vi "QueryServer_Template.vi"() -> ()   [LabVIEW 2019]
panel:
  in  "stop":bool
  in  "Server Address":string
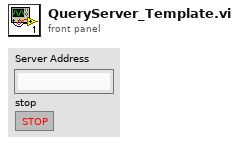
[diagram p1: front panel]
types:
  T1 = cluster{"event":refnum<user-event>, "event":refnum<user-event>, "event":refnum<user-event>}
  T2 = typedef "QueryServer_gRPCid.ctl" = cluster{"ID":u64}
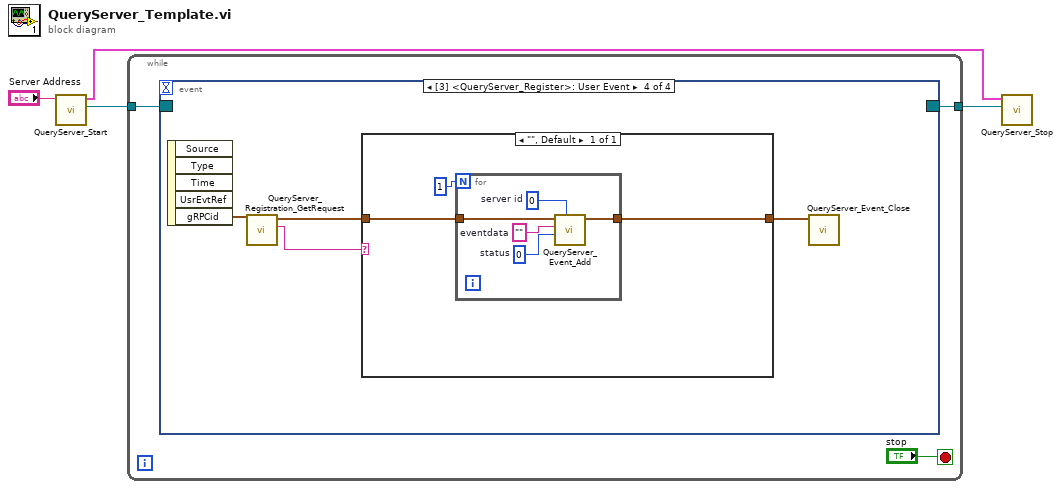
[diagram p0: block diagram]
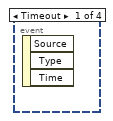
[diagram p2: hidden frame]
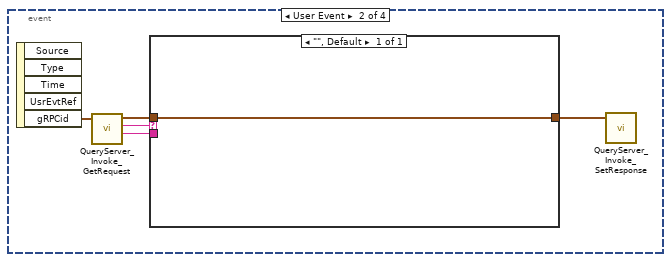
[diagram p3: hidden frame]
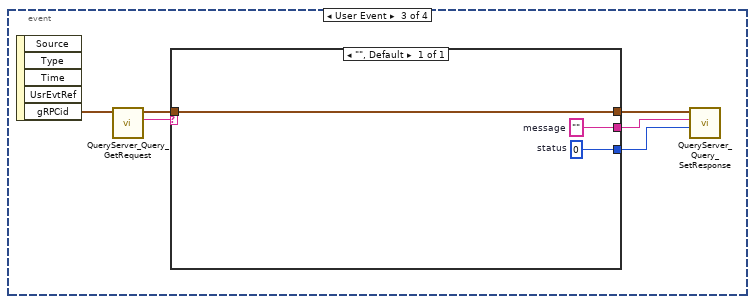
[diagram p4: hidden frame]
diagram:
  n1 = call "QueryServer_Start.vi"("Server Address"="Server Address") -> ("Event Registration Refnum"=w3:refnum<event-registration>, "Server Events"=w1:T1)  [unwired: 7 in, 1 out]
  n2 = while {
    tunnel: w3 -> [w6]
    tunnel: [w5] -> w2
    stop <- "stop" stop-if-true
    n3 = event shown="[3] <QueryServer_Register>: User Event" {
      selector: w6 -> [_ _ _ _]
      dyn-events: [_ _ _ _] -> w5
      timeout: _ -> [_ _ _ _]
      event Timeout {
        n4 = event-data() -> ()  [unwired: 1 in, 3 out]
      }
      event User Event {
        n5 = event-data() -> ("gRPCid"=w12:T2)  [unwired: 1 in, 4 out]
        n6 = call "QueryServer_Invoke_GetRequest.vi"("gRPCid"=w12) -> ("parameter"=w8:string, "command"=w11:string, "gRPCid out"=w10:T2)  [unwired: 5 in, 1 out]
        n7 = case shown="\"\", Default" w11 {
          tunnel: w10 -> [w13]
          tunnel: [w13] -> w9
          tunnel: w8 -> [_]
          frame "", Default {
          }
        }
        n8 = call "QueryServer_Invoke_SetResponse.vi"("gRPCid"=w9) -> ()  [unwired: 9 in, 1 out]
      }
      event User Event {
        n9 = event-data() -> ("gRPCid"=w19:T2)  [unwired: 1 in, 4 out]
        n10 = call "QueryServer_Query_GetRequest.vi"("gRPCid"=w19) -> ("gRPCid out"=w17:T2, "query"=w18:string)  [unwired: 7 in, 1 out]
        n11 = case shown="\"\", Default" w18 {
          tunnel: w17 -> [w22]
          tunnel: [w22] -> w16
          tunnel: [w21] -> w15
          tunnel: [w20] -> w14
          frame "", Default {
            w20 = 0  # status
            w21 = ""  # message
          }
        }
        n12 = call "QueryServer_Query_SetResponse.vi"("gRPCid"=w16, "message"=w15, "status"=w14) -> ()  [unwired: 7 in, 1 out]
      }
      event User Event {
        n13 = event-data() -> ("gRPCid"=w26:T2)  [unwired: 1 in, 4 out]
        n14 = call "QueryServer_Registration_GetRequest.vi"("gRPCid"=w26) -> ("gRPCid out"=w24:T2, "eventname"=w25:string)  [unwired: 7 in, 1 out]
        n15 = case shown="\"\", Default" w25 {
          tunnel: w24 -> [w29]
          tunnel: [w27] -> w23
          frame "", Default {
            n16 = for {
              N: 1 -> [_]
              tunnel: w29 -> [w34]
              tunnel: [w33] -> w27
              w30 = 0  # server id
              w31 = 0  # status
              w32 = ""  # eventdata
              n17 = call "QueryServer_Event_Add.vi"("server id"=w30, "status"=w31, "eventdata"=w32, "gRPCid"=w34) -> ("gRPCid out"=w33:T2)  [unwired: 6 in, 1 out]
            }
          }
        }
        n18 = call "QueryServer_Event_Close.vi"("gRPCid"=w23) -> ()  [unwired: 9 in, 1 out]
      }
    }
  }
  n19 = call "QueryServer_Stop.vi"("Server Events"=w1, "Event Registration Refnum"=w2) -> ()  [unwired: 8 in, 1 out]
